vi "ParseFile.vi"(8 "error in (no error)":errorcluster, 11 "FileContents":string) -> (0 "error out":errorcluster, 3 "Config":T1)   [LabVIEW 2017]
uses:
  <vilib>/WebServerConfig/Config.ctl
  <vilib>/WebServerConfig/Server.ctl
  <vilib>/WebServerConfig/Alias.ctl
  <vilib>/WebServerConfig/ErrorDocument.ctl
  <vilib>/WebServerConfig/Action.ctl
  <vilib>/WebServerConfig/Redirect.ctl
  <vilib>/WebServerConfig/Interface.ctl
  <vilib>/WebServerConfig/AddHandler.ctl
  <vilib>/WebServerConfig/SSL.ctl
  <vilib>/WebServerConfig/CustomLog.ctl
  <vilib>/WebServerConfig/LoadModule.ctl
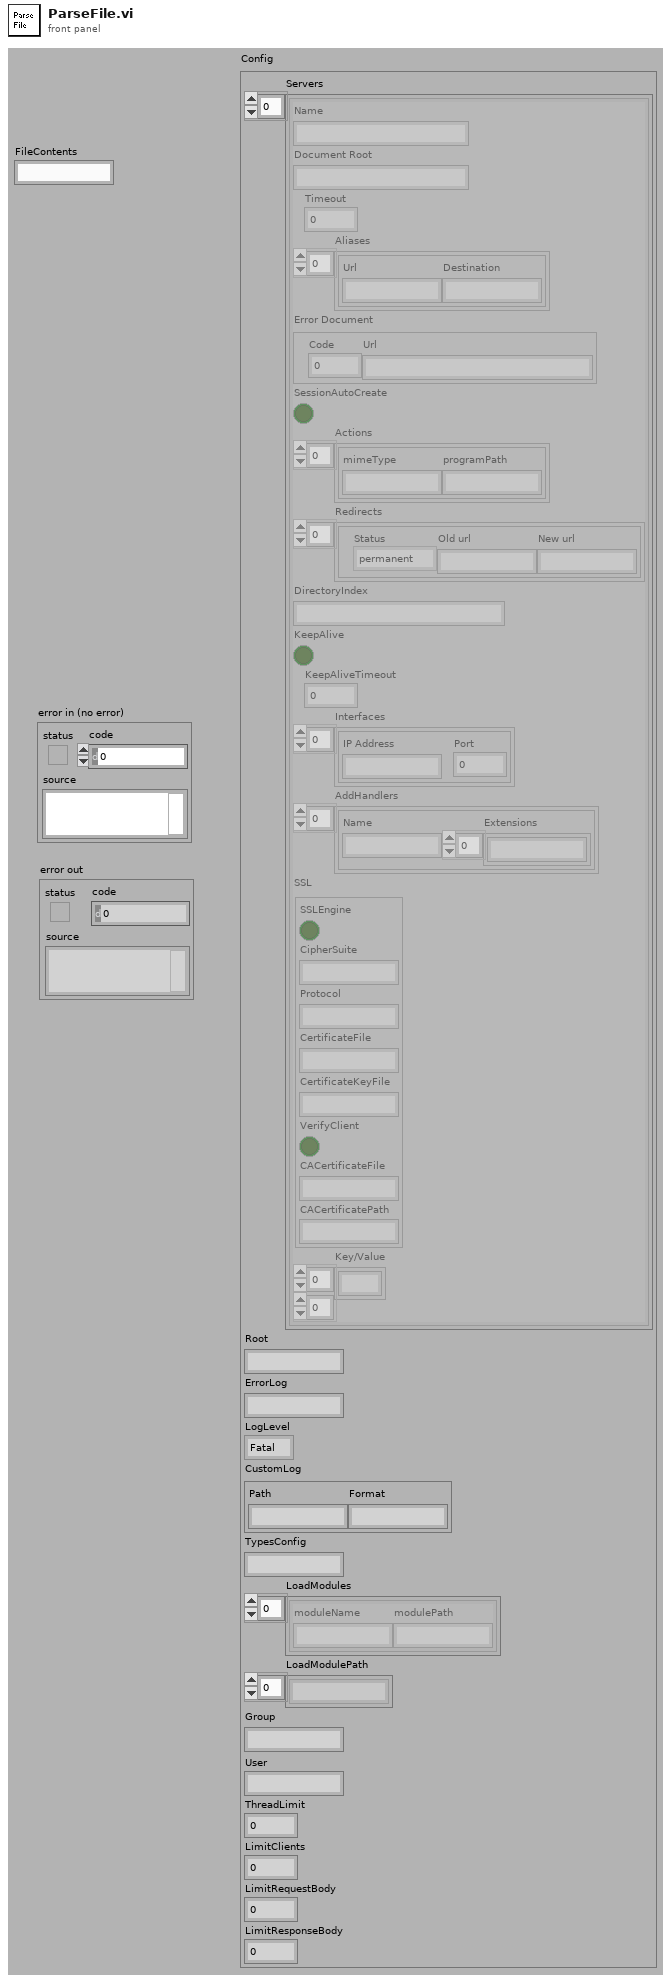
[diagram p1: front panel]
types:
  T1 = typedef "Config.ctl" = cluster{"Servers":T2[], "Root":string, "ErrorLog":string, "LogLevel":enum16{"Fatal", "Error", "Warn", "Info", "Debug", "5", "6", "7", "8", "Verbose"}, "CustomLog":T10, "TypesConfig":string, "LoadModules":T11[], "LoadModulePath":string[], "Group":string, "User":string, "ThreadLimit":u32, "LimitClients":u32, "LimitRequestBody":u32, "LimitResponseBody":u32}
  T2 = typedef "Server.ctl" = cluster{"Name":string, "Document Root":string, "Timeout":u32, "Aliases":T3[], "Error Document":T4, "SessionAutoCreate":bool, "Actions":T5[], "Redirects":T6[], "DirectoryIndex":string, "KeepAlive":bool, "KeepAliveTimeout":u32, "Interfaces":T7[], "AddHandlers":T8[], "SSL":T9, "Key/Value":string[][]}
  T3 = typedef "Alias.ctl" = cluster{"Url":string, "Destination":string}
  T4 = typedef "ErrorDocument.ctl" = cluster{"Code":u16, "Url":string}
  T5 = typedef "Action.ctl" = cluster{"mimeType":string, "programPath":string}
  T6 = typedef "Redirect.ctl" = cluster{"Status":enum16{"permanent", "temp", "seeother", "gone"}, "Old url":string, "New url":string}
  T7 = typedef "Interface.ctl" = cluster{"IP Address":string, "Port":u16}
  T8 = typedef "AddHandler.ctl" = cluster{"Name":string, "Extensions":string[]}
  T9 = typedef "SSL.ctl" = cluster{"SSLEngine":bool, "CipherSuite":string, "Protocol":string, "CertificateFile":string, "CertificateKeyFile":string, "VerifyClient":bool, "CACertificateFile":string, "CACertificatePath":string}
  T10 = typedef "CustomLog.ctl" = cluster{"Path":string, "Format":string}
  T11 = typedef "LoadModule.ctl" = cluster{"moduleName":string, "modulePath":string}
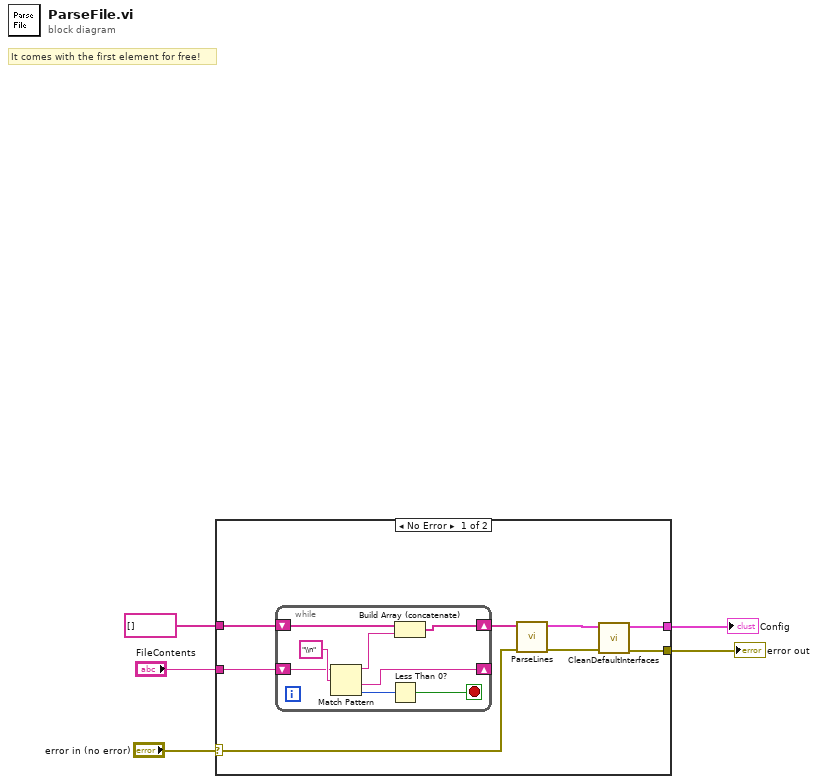
[diagram p0: block diagram]
diagram:
  # "It comes with the first element for free!"
  n1 = case shown="No Error" "error in (no error)" {
    selector: "error in (no error)" -> [w13 w22]
    tunnel: string[] [] -> [w10 _]
    tunnel: [w12 _] -> w4
    tunnel: [w11 w22] -> w3
    tunnel: "FileContents" -> [w9 _]
    frame No Error {
      n2 = while {
        shift-right: [w17] -> w6
        shift-left: w10 -> [w16]
        shift-right: [w15] -> _
        shift-left: w9 -> [w14]
        stop <- w19 stop-if-true
        n3 = Match Pattern(string=w14, regular expression="\\n") -> (before substring=w18:string, after substring=w15:string, offset past match=w20:i32)  [unwired: 1 in, 1 out]
        n4 = Less Than 0?(x=w20) -> (x < 0?=w19:bool)
        n5 = Build Array (concatenate)(w16, w18) -> (w17:string[])
      }
      n6 = call <vilib>:"ParseLines.vi"("error in"=w13, "Lines"=w6) -> ("error out"=w7:errorcluster, "Config"=w8:T1)  [unwired: 8 in]
      n7 = call <vilib>:"CleanDefaultInterfaces.vi"("error in"=w7, "Config in"=w8) -> ("error out"=w11:errorcluster, "Config out"=w12:T1)  [unwired: 8 in]
    }
    frame Error {
    }
  }
  "Config" <- w4
  "error out" <- w3
